vi "L298N_Driver.vi"() -> ()   [LabVIEW 2019]
uses:
  <vilib>/myRIO/Instrument Drivers/Onboard IO/DIO/DIO.lvlib
  L298N_Driver/L298N_Action_Enum.ctl
  L298N_Ref.ctl
panel:
  in  "L298N_Ref":T1
  in  "Action_Moteur":T2
  out "Error Out":errorcluster caption="Sortie d'erreur"
  in  "Error In":errorcluster caption="Entrée d'erreur"
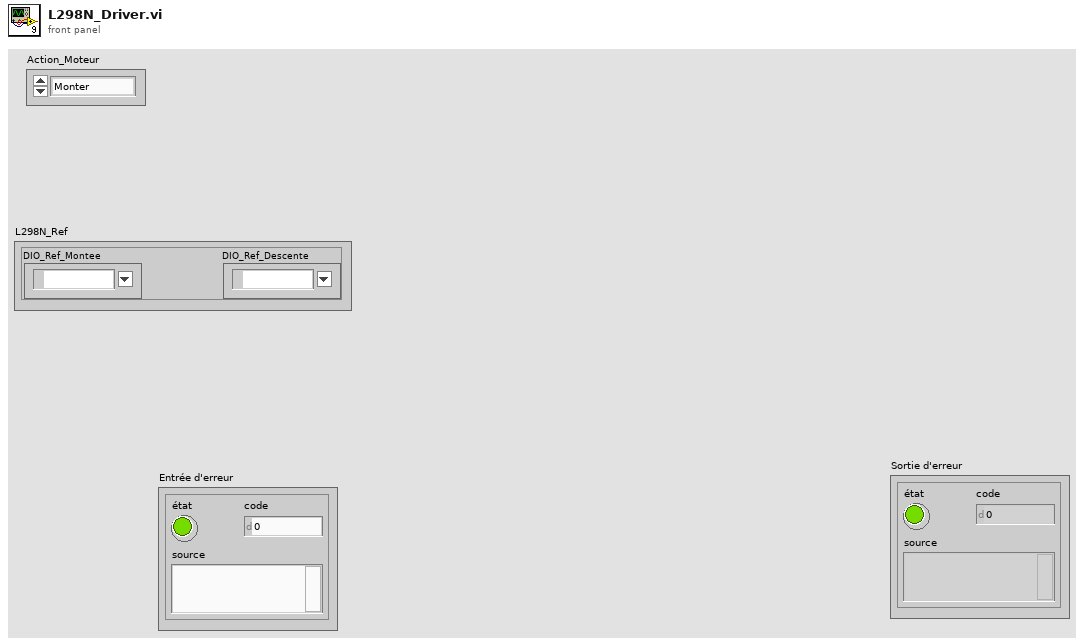
[diagram p1: front panel]
types:
  T1 = typedef "L298N_Ref.ctl" = cluster{"DIO_Ref_Montee":refnum<k21>, "DIO_Ref_Descente":refnum<k21>}
  T2 = typedef "L298N_Action_Enum.ctl" = enum16{"Monter", "Descendre", "Arreter"}
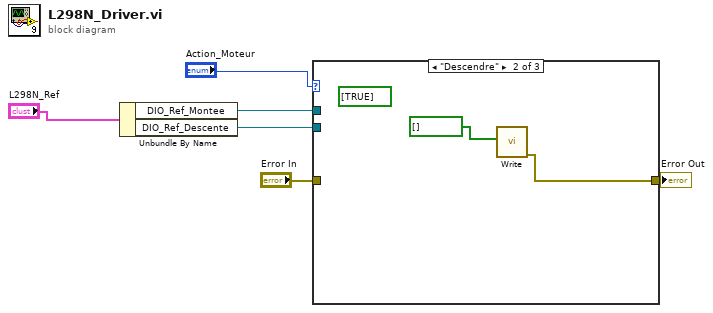
[diagram p0: block diagram]
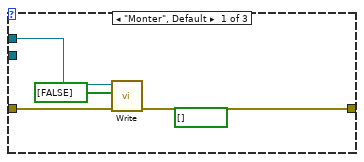
[diagram p2: hidden frame]
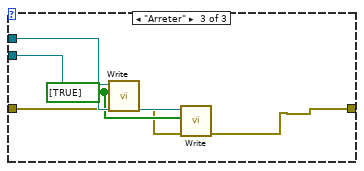
[diagram p3: hidden frame]
diagram:
  n1 = Unbundle By Name("L298N_Ref") -> ("DIO_Ref_Montee"=w3:refnum<k21>, "DIO_Ref_Descente"=w2:refnum<k21>)
  n2 = case shown="\"Descendre\"" "Action_Moteur" {
    tunnel: w2 -> [_ _ w18]
    tunnel: w3 -> [w8 _ w17]
    tunnel: "Error In" -> [w9 _ w15]
    tunnel: [w7 w11 w13] -> w5
    frame "Monter", Default {
      (unwired) bool[] [] ("Values")
      n3 = call <vilib>:"Write.vi"("error in (no error)"=w9, "Values"=bool[] [FALSE], "DIO Ref In"=w8) -> ("error out"=w7:errorcluster)  [unwired: 6 in, 1 out]
    }
    frame "Descendre" {
      (unwired) bool[] [TRUE] ("Values")
      n4 = call <vilib>:"Write.vi"("Values"=bool[] []) -> ("error out"=w11:errorcluster)  [unwired: 8 in, 1 out]
    }
    frame "Arreter" {
      w16 = bool[] [TRUE] ("Values")
      n5 = call <vilib>:"Write.vi"("error in (no error)"=w15, "Values"=w16, "DIO Ref In"=w18) -> ("error out"=w14:errorcluster)  [unwired: 6 in, 1 out]
      n6 = call <vilib>:"Write.vi"("error in (no error)"=w14, "Values"=w16, "DIO Ref In"=w17) -> ("error out"=w13:errorcluster)  [unwired: 6 in, 1 out]
    }
  }
  "Error Out" <- w5
